vi "Fetch Min Max Waveform [MmW].vi"(0 "CS++Scope":refnum<class "CS++Scope.lvclass">, 1 "channel name (\"CHANNEL1\")":string="CHANNEL1", 2 "waveform size (0)":i32=1000, 5 "error in (no error)":errorcluster) -> (11 "min waveform array":dbl[unit][](array[numeric]) format="%.3f", 13 "max waveform array":dbl[unit][](array[numeric]) format="%.3f", 14 "CS++Scope out":refnum<class "CS++Scope.lvclass">, 15 "actual points":i32, 16 "initial x":dbl[unit] format="%^.2e", 17 "x increment":dbl[unit] format="%^.2e", 19 "error out":errorcluster)   [LabVIEW 2016, in "CS++Scope.lvlib" / "CS++Scope.lvclass"]
doc: "This VI returns the minimum and maximum waveforms that the oscilloscope acquires for the channel you specify. If the channel is not enabled for the acquisition, this VI returns IVISCOPE_ERROR_CHANNEL_NOT_ENABLED (0xBFFA2001)error.\nThe waveforms are from an acquisition that you previously initiated. Use this VI to fetch waveforms when you set the acquisition type to IVISCOPE_VAL_PEAK_DETECT or IVISCOPE_VAL_ENVELOPE. If the acquisition type is not one of the listed types, the VI returns the IVISCOPE_ERROR_INVALID_ACQ_TYPE (0xBFFA2004) error.\n\nUse the IviScope Initiate Acquisition VI to start an acquisition on the channels that you enable with the IviScope Configure Channel VI. The oscilloscope acquires the min/max waveforms for the enabled channels concurrently. You use the IviScope Acquisition Status VI to determine when the acquisition is complete. You must call this VI separately for each enabled channel to obtain the min/max waveforms.\nYou can call the IviScope Read Min Max Waveform [MmW] VI instead of the IviScope Initiate Acquisition VI. The IviScope Read Min Max Waveform [MmW] VI starts an acquisition on all enabled channels, waits for the acquisition to complete, and returns the min/max waveforms for the channel you specify. You call this VI to obtain the min/max waveforms for each of the remaining channels.\n\nNotes:\n(1) After this VI executes, each element in the Min Waveform Array and Max Waveform Array parameters is either a voltage or a value indicating that the oscilloscope could not sample a voltage.\n\n(2) You configure the interpolation method the oscilloscope uses with the IviScope Is Invalid Waveform Element VI. If you disable interpolation, the oscilloscope does not interpolate points in the waveform. If the oscilloscope cannot sample a value for a point in the waveform, the driver sets the corresponding element in the Waveform Array to an IEEE defined NaN (Not a Number) value and the VI returns IVISCOPE_WARN_INVALID_WFM_ELEMENT (0x3FFA2001). \n\n(3) You can test a waveform value for an invalid value condition by calling the IviScope Is Invalid Waveform Element VI.\n\n(4) This VI does not check the instrument status. Typically, you call this VI only in a sequence of calls to other low-level driver VIs. The sequence performs one operation. You use the low-level VIs to optimize one or more aspects of interaction with the instrument. If you want to check the instrument status, call the IviScope Error-Query VI at the conclusion of the sequence.\n\n(5) The class driver returns a simulated minimum and maximum waveform when this VI is called and the IviScope>>Inherent IVI Settings>>User Options>>Simulate property is set to TRUE and the IviScope>>Inherent IVI Settings>>User Options>>Use Specific Simulation property is set to FALSE. For information on how to configure a simulated waveform, refer to the online help manual.\n\n(6) This VI is part of the IviScopeMinMaxWaveform [MmW] extension group."
uses:
  CS++Scope.lvclass
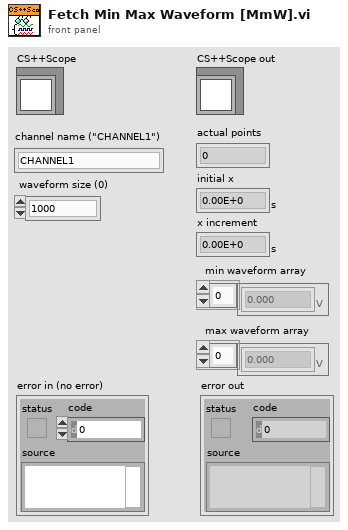
[diagram p1: front panel]
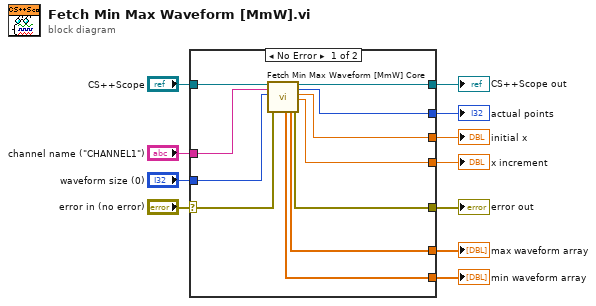
[diagram p0: block diagram]
diagram:
  n1 = case shown="No Error" "error in (no error)" {
    selector: "error in (no error)" -> [w21 w24]
    tunnel: [w20 w24] -> w10
    tunnel: [w19 w23] -> w7
    tunnel: "CS++Scope" -> [w22 w23]
    tunnel: "channel name (\"CHANNEL1\")" -> [w17 _]
    tunnel: "waveform size (0)" -> [w18 _]
    tunnel: [w16 _] -> w5
    tunnel: [w15 _] -> w4
    tunnel: [w14 _] -> w3
    tunnel: [w13 _] -> w2
    tunnel: [w12 _] -> w1
    frame No Error {
      n2 = call-dynamic "Fetch Min Max Waveform [MmW] Core.vi"("CS++Scope"=w22, "channel name (\"CHANNEL1\")"=w17, "waveform size (0)"=w18, "error in (no error)"=w21) -> ("min waveform array"=w15:dbl[unit][], "max waveform array"=w16:dbl[unit][], "CS++Scope out"=w19:refnum<class "CS++Scope.lvclass">, "actual points"=w12:i32, "initial x"=w13:dbl[unit], "x increment"=w14:dbl[unit], "error out"=w20:errorcluster)  [unwired: 9 in]
    }
    frame Error {
    }
  }
  "error out" <- w10
  "actual points" <- w1
  "initial x" <- w2
  "x increment" <- w3
  "min waveform array" <- w4
  "max waveform array" <- w5
  "CS++Scope out" <- w7
